vi "21414111邱致綸.vi"() -> ()   [LabVIEW 2017]
panel:
  out "埃":dbl
  out "­¼":dbl
  out "搭":dbl
  out "¥[":dbl
  in  "y":dbl
  in  "x":dbl
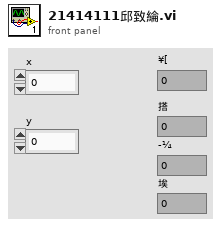
[diagram p1: front panel]
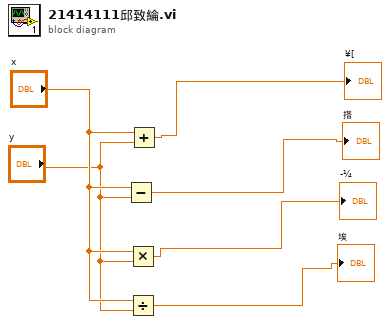
[diagram p0: block diagram]
diagram:
  n1 = Subtract(x="x", y="y") -> (x-y=→"搭":dbl)
  n2 = Multiply(x="x", y="y") -> (x*y=→"­¼":dbl)
  n3 = Divide(x="x", y="y") -> (x/y=→"埃":dbl)
  n4 = Add(x="x", y="y") -> (x+y=→"¥[":dbl)
